vi "PID.vi"(8 "error in (no error)":errorcluster, 9 "Process Variable":dbl, 10 "Setpoint":dbl, 11 "PID in":refnum<class "PID.lvclass">) -> (0 "error out":errorcluster, 3 "PID out":refnum<class "PID.lvclass">)   [LabVIEW 2024, in "PID.lvlib" / "PID.lvclass"]
uses:
  PID.lvclass
panel:
  out "Output":dbl
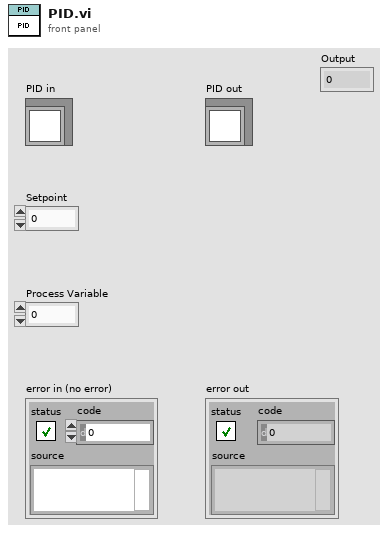
[diagram p1: front panel]
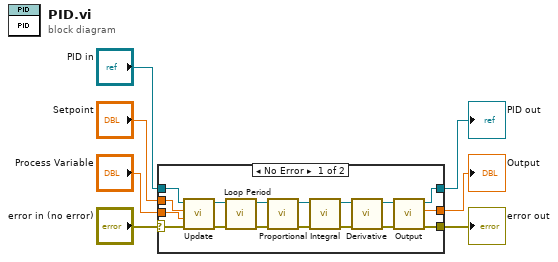
[diagram p0: block diagram]
diagram:
  n1 = case shown="No Error" "error in (no error)" {
    selector: "error in (no error)" -> [w15 w26]
    tunnel: [w10 w26] -> w6
    tunnel: [w8 w25] -> w4
    tunnel: "PID in" -> [w16 w25]
    tunnel: "Setpoint" -> [w14 _]
    tunnel: "Process Variable" -> [w13 _]
    tunnel: [w9 _] -> w1
    frame No Error {
      n2 = call-dynamic "Update.vi"("error in (no error)"=w15, "Process Variable"=w13, "Setpoint"=w14, "PID in"=w16) -> ("error out"=w19:errorcluster, "PID out"=w20:refnum<class "PID.lvclass">)  [unwired: 6 in]
      n3 = call-dynamic "Loop Period.vi"("error in (no error)"=w19, "PID in"=w20) -> ("error out"=w17:errorcluster, "PID out"=w18:refnum<class "PID.lvclass">)  [unwired: 8 in]
      n4 = call-dynamic "Proportional.vi"("error in (no error)"=w17, "PID in"=w18) -> ("error out"=w23:errorcluster, "PID out"=w24:refnum<class "PID.lvclass">)  [unwired: 8 in]
      n5 = call-dynamic "Integral.vi"("error in (no error)"=w23, "PID in"=w24) -> ("error out"=w21:errorcluster, "PID out"=w22:refnum<class "PID.lvclass">)  [unwired: 8 in]
      n6 = call-dynamic "Derivative.vi"("error in (no error)"=w21, "PID in"=w22) -> ("error out"=w11:errorcluster, "PID out"=w12:refnum<class "PID.lvclass">)  [unwired: 8 in]
      n7 = call-dynamic "Output.vi"("error in (no error)"=w11, "PID in"=w12) -> ("error out"=w10:errorcluster, "Output"=w9:dbl, "PID out"=w8:refnum<class "PID.lvclass">)  [unwired: 7 in]
    }
    frame Error {
    }
  }
  "error out" <- w6
  "PID out" <- w4
  "Output" <- w1
